vi "ElevatorDashReadInnerNetwork.vi"() -> (0 "Stage3HighLimitSwitch":bool, 1 "Stage3MotorOutput":dbl, 2 "Stage3PositionHeight":dbl, 3 "Stage3PosDemandHeight":dbl, 4 "Stage3LowLimitSwitch":bool, 5 "Stage3LowWristClampActive":bool, 6 "Stage3OnTarget":bool)   [LabVIEW 2023]
uses:
  <vilib>/Rock Robotics/Network Tables/NT Read Number.vi
  <vilib>/Rock Robotics/Network Tables/NT Read Boolean.vi
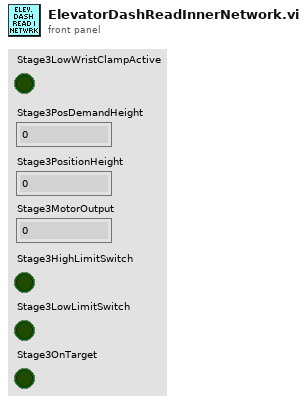
[diagram p1: front panel]
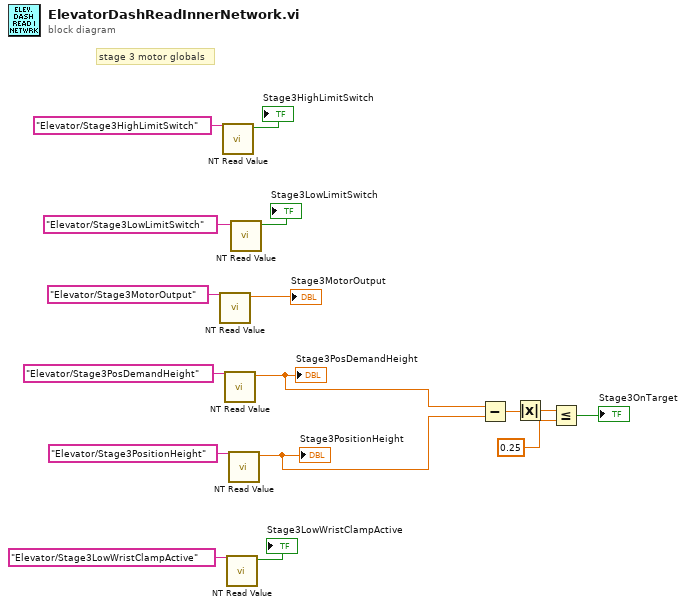
[diagram p0: block diagram]
diagram:
  # "stage 3 motor globals"
  n1 = call-poly <vilib>:"NT Read Value.vi"("name"="Elevator/Stage3MotorOutput") -> ("value"=→"Stage3MotorOutput":dbl)  [unwired: 8 in, 2 out]
  n2 = call-poly <vilib>:"NT Read Value.vi"("name"="Elevator/Stage3HighLimitSwitch") -> ("value"=→"Stage3HighLimitSwitch":bool)  [unwired: 8 in, 2 out]
  n3 = call-poly <vilib>:"NT Read Value.vi"("name"="Elevator/Stage3PosDemandHeight") -> ("value"=w8:dbl)  [unwired: 8 in, 2 out]
  "Stage3PosDemandHeight" <- w8
  n4 = call-poly <vilib>:"NT Read Value.vi"("name"="Elevator/Stage3LowWristClampActive") -> ("value"=→"Stage3LowWristClampActive":bool)  [unwired: 8 in, 2 out]
  n5 = call-poly <vilib>:"NT Read Value.vi"("name"="Elevator/Stage3PositionHeight") -> ("value"=w7:dbl)  [unwired: 8 in, 2 out]
  "Stage3PositionHeight" <- w7
  n6 = call-poly <vilib>:"NT Read Value.vi"("name"="Elevator/Stage3LowLimitSwitch") -> ("value"=→"Stage3LowLimitSwitch":bool)  [unwired: 8 in, 2 out]
  n7 = Subtract(x=w8, y=w7) -> (x-y=w6:dbl)
  n8 = Absolute Value(x=w6) -> (abs(x)=w5:dbl)
  n9 = Less Or Equal?(x=w5, y=0.25) -> (x <= y?=→"Stage3OnTarget":bool)
